vi "scaleexposure.vi"(9 "black":i32, 10 "white":i32, 11 "image in":u16[][](array[numeric])) -> (3 "image out":u16[][](array[numeric]))   [LabVIEW 2017]
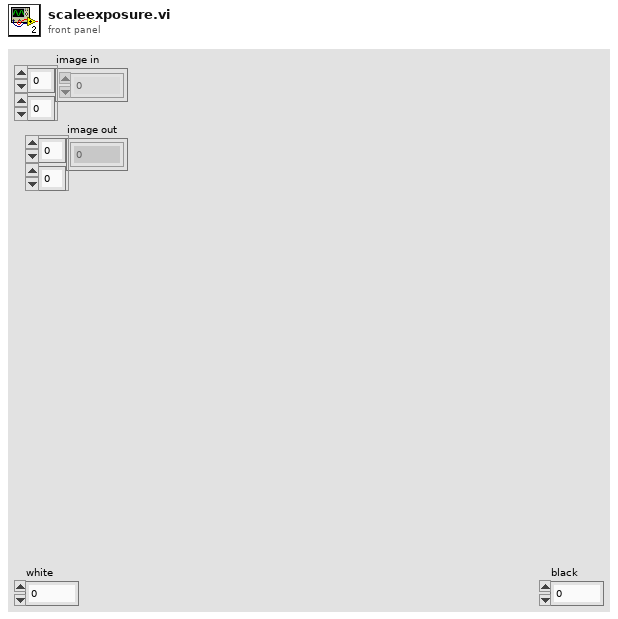
[diagram p1: front panel]
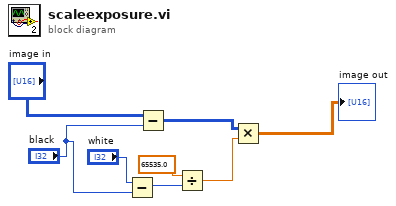
[diagram p0: block diagram]
diagram:
  n1 = Subtract(x="white", y="black") -> (x-y=w5:i32)
  n2 = Subtract(x="image in", y="black") -> (x-y=w4:i32[][])
  n3 = Divide(x=65535.0, y=w5) -> (x/y=w3:dbl)
  n4 = Multiply(x=w4, y=w3) -> (x*y=→"image out":dbl[][])
